vi "Write panel message (SubVI).vi"(4 "rpm":refnum<vi>, 5 "rpm":bool, 6 "PrintTime":bool=TRUE, 7 "Stop":refnum<vi>, 8 "error in (no error)":errorcluster, 9 "Time to wait":dbl, 10 "Strin":string, 11 "String in":refnum<vi>) -> (0 "error out":errorcluster)   [LabVIEW 2017]
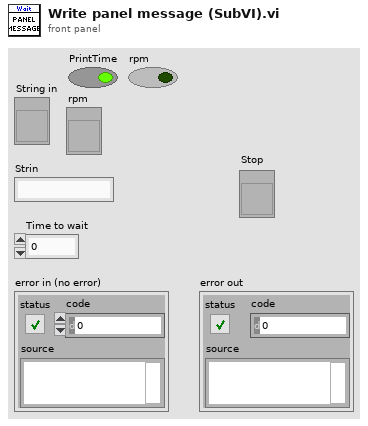
[diagram p1: front panel]
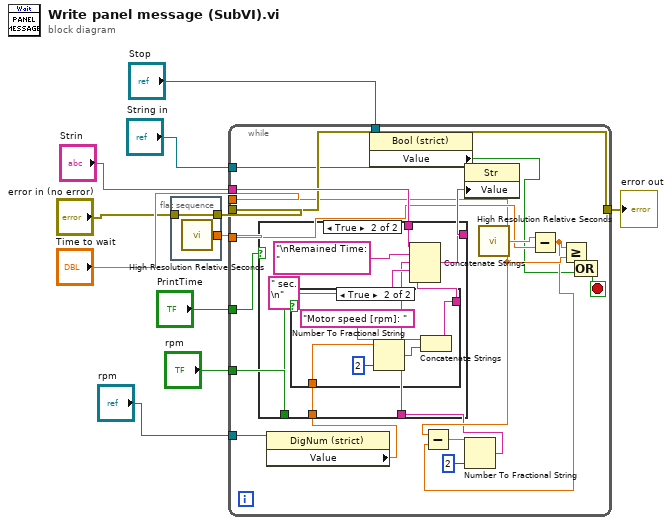
[diagram p0: block diagram]
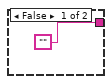
[diagram p3: hidden frame]
diagram:
  n1 = flat-sequence {
    tunnel: [w13] -> w7
    tunnel: "error in (no error)" -> [w13]
    tunnel: [w12] -> w8
    frame #0 {
      n2 = call <vilib>:"High Resolution Relative Seconds.vi"() -> ("relative seconds"=w12:dbl)
    }
  }
  n3 = while {
    tunnel: "Strin" -> [w32]
    tunnel: w7 -> [w27]
    tunnel: w8 -> [w29]
    tunnel: "Time to wait" -> [w23]
    tunnel: [w27] -> w10
    tunnel: "String in" -> [w26]
    tunnel: "Stop" -> [w20]
    tunnel: "PrintTime" -> [w17]
    tunnel: "rpm" -> [w16]
    tunnel: "rpm" -> [w15]
    stop <- w19 stop-if-true
    n4 = property class="DigNum (strict)"(reference=w15) -> ("Value"=w14:dbl)  [unwired: 1 in, 2 out]
    n5 = property class="Bool (strict)"(reference=w20) -> ("Value"=w18:bool)  [unwired: 1 in, 2 out]
    n6 = call <vilib>:"High Resolution Relative Seconds.vi"() -> ("relative seconds"=w30:dbl)
    n7 = Subtract(x=w30, y=w29) -> (x-y=w22:dbl)
    n8 = Subtract(x=w23, y=w22) -> (x-y=w24:dbl)
    n9 = Number To Fractional String(number=w24, precision (6)=i16 2) -> (F-format string=w21:string)  [unwired: 2 in]
    n10 = case shown="True" w17 {
      tunnel: w32 -> [w33 w41]
      tunnel: [w33 w38] -> w31
      tunnel: w21 -> [_ w37]
      tunnel: w16 -> [_ w36]
      tunnel: w14 -> [_ w34]
      frame False {
      }
      frame True {
        n11 = case shown="True" w36 {
          tunnel: ["" w44] -> w35
          tunnel: w34 -> [_ w43]
          frame False {
          }
          frame True {
            n12 = Number To Fractional String(number=w43, precision (6)=i16 2) -> (F-format string=w45:string)  [unwired: 2 in]
            n13 = Concatenate Strings("Motor speed [rpm]: " ("string"), w45) -> (w44:string)
          }
        }
        n14 = Concatenate Strings(w41, "\nRemained Time: " ("string"), w37, " sec.\n" ("string"), w35) -> (w38:string)
      }
    }
    n15 = property class="Str"(reference=w26, "Value"=w31) -> ()  [unwired: 1 in, 2 out]
    n16 = Greater Or Equal?(x=w22, y=w23) -> (x >= y?=w28:bool)
    n17 = Compound Arithmetic op=OR(w28, w18) -> (w19:bool)
  }
  "error out" <- w10
